vi "Get Cell .NET.vi"(11 "Cell in":refnum<class "Cell.lvclass">) -> (2 "Cell .NET":refnum<k24>, 3 "Cell out":refnum<class "Cell.lvclass">)   [LabVIEW 2023, in "SourceGrid.lvlib" / "Cell.lvclass"]
uses:
  Cell.lvclass
  D:/git/Sourcegrid-LabVIEW/dll/SourceGrid.dll
  dll/SourceGrid.dll
  Cell.lvclass/Cell.ctl
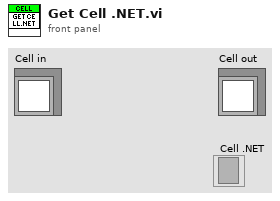
[diagram p1: front panel]
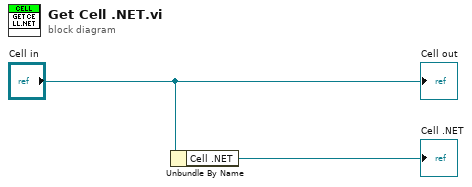
[diagram p0: block diagram]
diagram:
  n1 = Unbundle By Name("Cell in") -> ("Cell .NET"=→"Cell .NET":refnum<k24>)
  "Cell out" <- "Cell in"
